vi "Write Reference.vi"(8 "error in (no error)":errorcluster, 10 "Reference":refnum<vi>, 11 "Chart in":refnum<class "Chart.lvclass">) -> (0 "error out":errorcluster, 3 "Chart out":refnum<class "Chart.lvclass">)   [LabVIEW 2024, in "Chart.lvclass"]
uses:
  Chart.lvclass
  Chart.lvclass/Chart.ctl
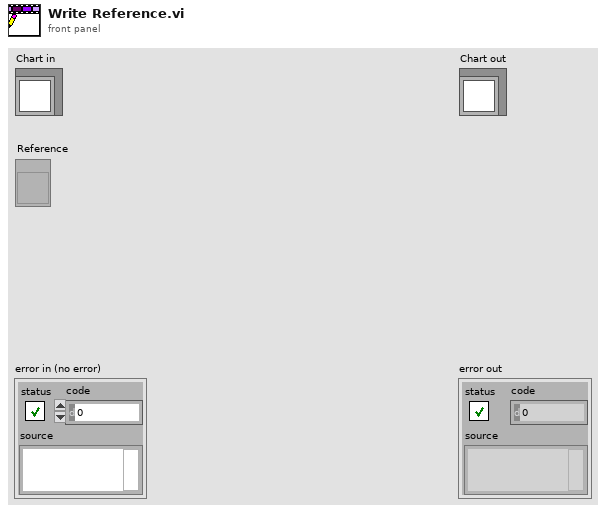
[diagram p1: front panel]
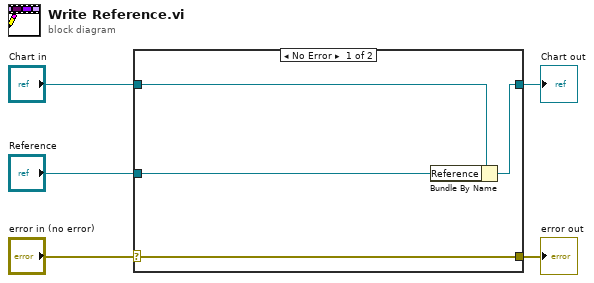
[diagram p0: block diagram]
diagram:
  n1 = case shown="No Error" "error in (no error)" {
    selector: "error in (no error)" -> [w9 w10]
    tunnel: [w9 w10] -> w4
    tunnel: [w7 w11] -> w2
    tunnel: "Chart in" -> [w8 w11]
    tunnel: "Reference" -> [w6 _]
    frame No Error {
      n2 = Bundle By Name(cluster=w8, "Reference"=w6) -> (w7:refnum<class "Chart.lvclass">)
    }
    frame Error {
    }
  }
  "error out" <- w4
  "Chart out" <- w2
